vi "Execute.vi"(8 "error in (no error)":errorcluster, 9 "System in":refnum<class "System.lvclass">, 10 "Command in":refnum<class "Command.lvclass">, 11 "CT-Energized-State in":refnum<class "CT-Energized-State.lvclass">) -> (0 "error out":errorcluster, 2 "Next State":refnum<class "State.lvclass">, 3 "CT-Energized-State out":refnum<class "CT-Energized-State.lvclass">)   [LabVIEW 2013, in "CT-Energized-State.lvclass"]
uses:
  CT-Energized-State.lvclass
  Commands/Command/Command.lvclass
  Systems/System/System.lvclass
  State/State.lvclass
  Systems/Catapult/Catapult.lvclass
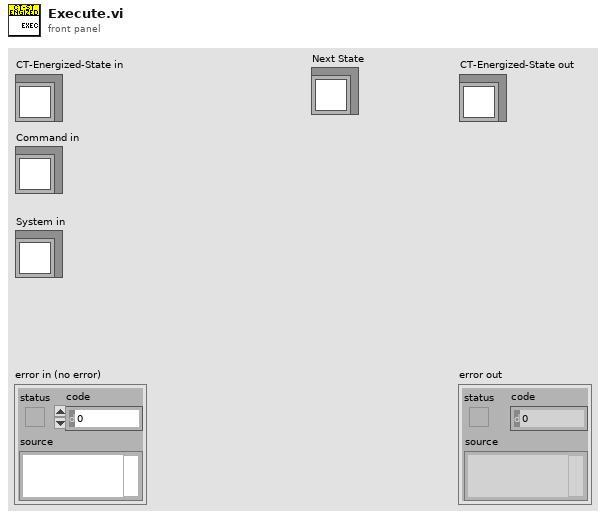
[diagram p1: front panel]
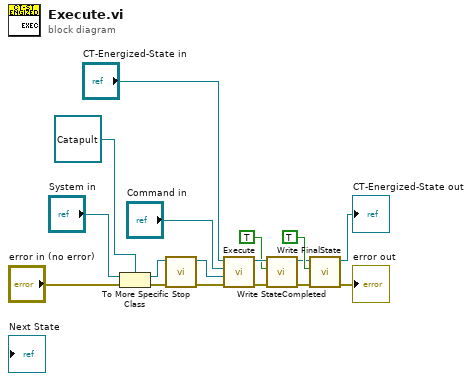
[diagram p0: block diagram]
diagram:
  n1 = To More Specific Class(target class=refnum<class "Catapult.lvclass"> refnum ("Catapult.lvclass"), reference="System in", error in="error in (no error)") -> (specific class reference=w12:refnum<class "Catapult.lvclass">, error out=w11:errorcluster)
  n2 = call-dynamic "Stop.vi"("error in (no error)"=w11, "Catapult in"=w12) -> ("error out"=w10:errorcluster, "Catapult out"=w9:refnum<class "Catapult.lvclass">)  [unwired: 8 in]
  n3 = call-parent "Execute.vi"("error in (no error)"=w10, "System in"=w9, "Command in"="Command in", "State in"="CT-Energized-State in") -> ("error out"=w2:errorcluster, "State out"=w5:refnum<class "CT-Energized-State.lvclass">)  [unwired: 5 in, 1 out]
  n4 = call-dynamic "Write StateCompleted.vi"("error in (no error)"=w2, "StateCompleted"=TRUE, "State in"=w5) -> ("error out"=w1:errorcluster, "State out"=w4:refnum<class "CT-Energized-State.lvclass">)  [unwired: 7 in]
  n5 = call-dynamic "Write FinalState.vi"("error in (no error)"=w1, "FinalState"=TRUE, "State in"=w4) -> ("error out"=→"error out":errorcluster, "State out"=→"CT-Energized-State out":refnum<class "CT-Energized-State.lvclass">)  [unwired: 7 in]
